vi "VI_read.vi"(8 "error in (no error)":errorcluster, 11 "File bytestream":string) -> (0 "error out":errorcluster, 2 "Resource type":string, 3 "Blocks":T1(c390), 4 "Icon":picture, 5 "Version":T2)   [LabVIEW 2023]
uses:
  <vilib>/Utility/error.llb/Error Cluster From Error Code.vi
  <vilib>/ErrorRing/Error Ring.xnode
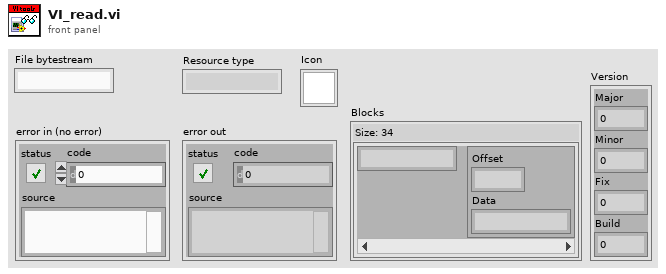
[diagram p1: front panel]
types:
  T1 = map{string, cluster{"Offset":i32, "Data":string}}
  T2 = cluster{"Major":u8, "Minor":u8, "Fix":u8, "Build":u8}
  T3 = cluster{"Int1":u32, "Int2":u32, "Int3":u32, "Offset":u32, "Size":u32}
  T4 = cluster{"RSRC_Identifier":u64, "RSRC_Type":u32, "RSRC_Creator":u32, "Info_Offset":u32, "Info_Size":u32, "Data_Offset":u32, "Data_Size":u32}
  T5 = cluster{"Version":cluster{"Major":u8, "Minor":u8, "Fix":u8, "Build":u8}, "Stage":enum8{"Development", "Alpha", "Beta", "Release"}, "Flags":u16, "VersionString":string, "VersionInfo":string}
  T6 = typedef "imagedata.ctl" = cluster{"image type":i32, "image depth":i32, "image":u8[], "mask":u8[], "colors":u32[], "Rectangle":cluster{"left":i16, "top":i16, "right":i16, "bottom":i16}}
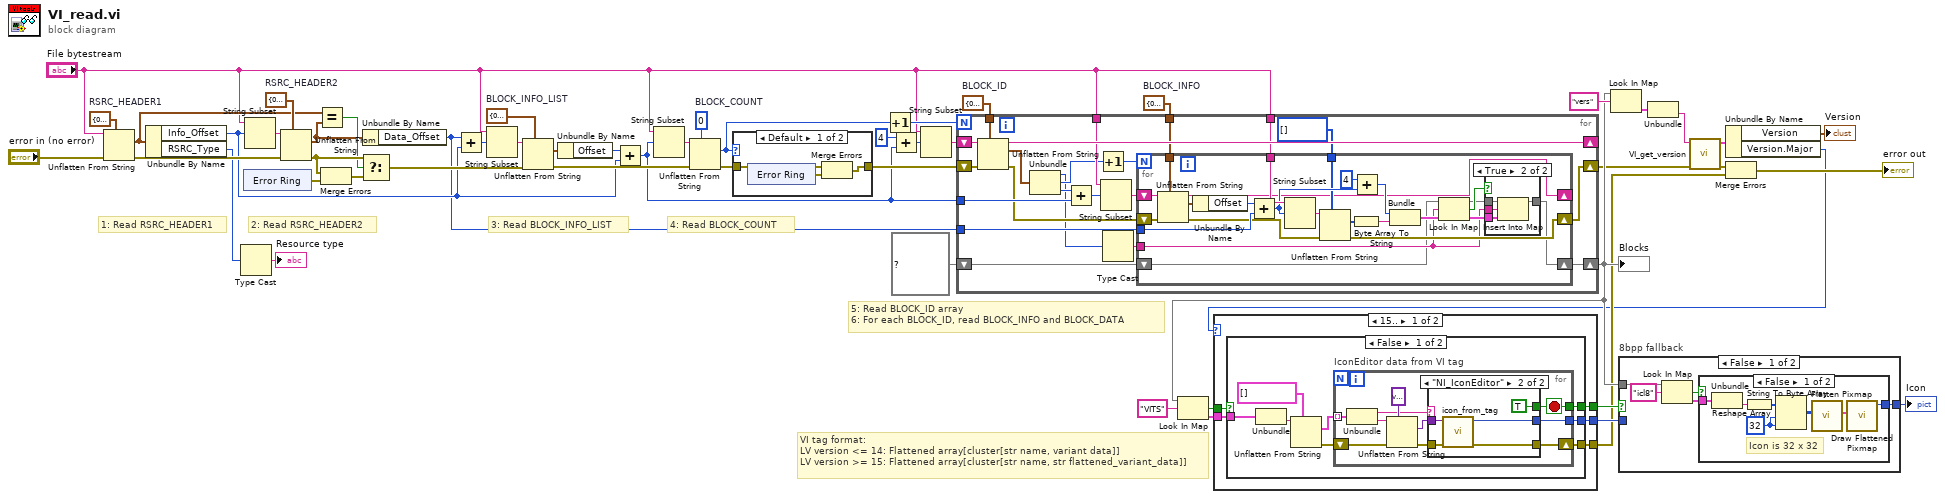
[diagram p0: block diagram]
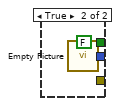
[diagram p3: hidden frame]
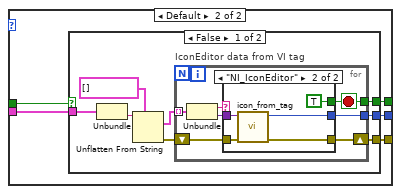
[diagram p4: hidden frame]
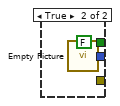
[diagram p6: hidden frame]
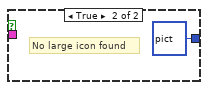
[diagram p7: hidden frame]
diagram:
  w25 = T3 {"Int1"=0, "Int2"=0, "Int3"=0, "Offset"=0, "Size"=0}  # BLOCK_INFO
  w33 = cluster{"Name":u32, "Count":u32, "Offset":u32} {"Name"=0, "Count"=0, "Offset"=0}  # BLOCK_ID
  w37 = 0  # BLOCK_COUNT
  w45 = T3 {"Int1"=0, "Int2"=0, "Int3"=0, "Offset"=0, "Size"=0}  # BLOCK_INFO_LIST
  w47 = T4 {"RSRC_Identifier"=0, "RSRC_Type"=0, "RSRC_Creator"=0, "Info_Offset"=0, "Info_Size"=0, "Data_Offset"=0, "Data_Size"=0}  # RSRC_HEADER2
  w53 = T4 {"RSRC_Identifier"=0, "RSRC_Type"=0, "RSRC_Creator"=0, "Info_Offset"=0, "Info_Size"=0, "Data_Offset"=0, "Data_Size"=0}  # RSRC_HEADER1
  # "VI tag format:\nLV version <= 14: Flattened array[cluster[str name, variant data]]\nLV version >= 15: Flattened array[cluster[str name, str flattened_variant_data]]"
  # "5: Read BLOCK_ID array\n6: For each BLOCK_ID, read BLOCK_INFO and BLOCK_DATA"
  # "4: Read BLOCK_COUNT"
  # "3: Read BLOCK_INFO_LIST"
  # "2: Read RSRC_HEADER2"
  # "1: Read RSRC_HEADER1"
  n1 = Unflatten From String(type=w53, binary string="File bytestream", error in (no error)="error in (no error)") -> (value=w40:T4, error out=w46:errorcluster)  [unwired: 2 in, 1 out]
  n2 = Unbundle By Name(w40) -> ("Info_Offset"=w28:u32, "RSRC_Type"=w20:u32)
  n3 = Type Cast(x=w20) -> (*(type *) &x=→"Resource type":string)  [unwired: 1 in]
  n4 = xnode "Error Ring"() -> ("error out"=w49:errorcluster)
  n5 = String Subset(string="File bytestream", offset (0)=w28) -> (substring=w48:string)  [unwired: 1 in]
  n6 = Unflatten From String(type=w47, binary string=w48, error in (no error)=w46) -> (value=w41:T4, error out=w52:errorcluster)  [unwired: 2 in, 1 out]
  n7 = Equal?(x=w40, y=w41) -> (x = y?=w50:bool)
  n8 = Merge Errors(w52, w49) -> (w51:errorcluster)
  n9 = Select(t=w52, s=w50, f=w51) -> (s? t:f=w42:errorcluster)
  n10 = Unbundle By Name(w41) -> ("Data_Offset"=w24:u32)
  n11 = Add(x=w24, y=w28) -> (x+y=w44:u32)
  n12 = String Subset(string="File bytestream", offset (0)=w44) -> (substring=w43:string)  [unwired: 1 in]
  n13 = Unflatten From String(type=w45, binary string=w43, error in (no error)=w42) -> (value=w35:T3, error out=w34:errorcluster)  [unwired: 2 in, 1 out]
  n14 = Unbundle By Name(w35) -> ("Offset"=w29:u32)
  n15 = Add(x=w29, y=w28) -> (x+y=w22:u32)
  n16 = String Subset(string="File bytestream", offset (0)=w22) -> (substring=w36:string)  [unwired: 1 in]
  n17 = Unflatten From String(type=w37, binary string=w36, error in (no error)=w34) -> (value=w38:i32, error out=w39:errorcluster)  [unwired: 2 in, 1 out]
  n18 = case "Valid Block Count?" shown="Default" w38 {
    tunnel: w39 -> [w55 w61]
    tunnel: [w54 w61] -> w30
    frame Default {
      n19 = xnode "Error Ring"() -> ("error out"=w56:errorcluster)
      n20 = Merge Errors(w55, w56) -> (w54:errorcluster)
    }
    frame 0..1000 {
      # "Valid block count"
    }
  }
  n21 = Increment(x=w38) -> (x+1=w31:i32)
  n22 = Add(x=u32 4 ("value"), y=w22) -> (x+y=w26:u32)
  n23 = String Subset(string="File bytestream", offset (0)=w26) -> (substring=w32:string)  [unwired: 1 in]
  n24 = for {
    N: w31 -> [_]
    shift-right: [w81] -> _
    shift-left: w32 -> [w83]
    tunnel: w33 -> [w82]
    shift-right: [w64] -> w5
    shift-left: w30 -> [w80]
    tunnel: w22 -> [w76]
    tunnel: "File bytestream" -> [w75]
    tunnel: w25 -> [w70]
    tunnel: w24 -> [w69]
    tunnel: "File bytestream" -> [w68]
    shift-right: [w62] -> w6
    shift-left: T1 {} ("map") -> [w63]
    n25 = Unflatten From String(type=w82, binary string=w83, error in (no error)=w80) -> (rest of the binary string=w81:string, value=w74:cluster{"Name":u32, "Count":u32, "Offset":u32}, error out=w71:errorcluster)  [unwired: 2 in]
    n26 = Unbundle(w74) -> ("Name"=w67:u32, "Count"=w73:u32, "Offset"=w72:u32)
    n27 = Add(x=w72, y=w76) -> (x+y=w77:u32)
    n28 = Increment(x=w73) -> (x+1=w79:u32)
    n29 = String Subset(string=w75, offset (0)=w77) -> (substring=w78:string)  [unwired: 1 in]
    n30 = Type Cast(x=w67) -> (*(type *) &x=w66:string)  [unwired: 1 in]
    n31 = for {
      N: w79 -> [_]
      shift-right: [w85] -> _
      shift-left: w78 -> [w106]
      shift-right: [w96] -> w64
      shift-left: w71 -> [w105]
      tunnel: w70 -> [w104]
      tunnel: w69 -> [w103]
      tunnel: w68 -> [w97]
      tunnel: u8[] [] -> [w93]
      tunnel: w66 -> [w87]
      shift-right: [w84] -> w62
      shift-left: w63 -> [w86]
      n32 = Unflatten From String(type=w104, binary string=w106, error in (no error)=w105) -> (rest of the binary string=w85:string, value=w102:T3, error out=w98:errorcluster)  [unwired: 2 in]
      n33 = Unbundle By Name(w102) -> ("Offset"=w101:u32)
      n34 = Add(x=w101, y=w103) -> (x+y=w94:u32)
      n35 = String Subset(string=w97, offset (0)=w94) -> (substring=w100:string)  [unwired: 1 in]
      n36 = Unflatten From String(type=w93, binary string=w100, error in (no error)=w98) -> (value=w99:u8[], error out=w96:errorcluster)  [unwired: 2 in, 1 out]
      n37 = Byte Array To String(unsigned byte array=w99) -> (string=w92:string)
      n38 = Add(x=u32 4 ("value"), y=w94) -> (x+y=w91:u32)
      n39 = Bundle(w91, "string"=w92) -> (w89:cluster{u32, "string":string})  [unwired: 1 in]
      n40 = Look In Map(map=w86, key=w87, default value=w89) -> (key not found?=w90:bool, value=w88:cluster{"Offset":i32, "Data":string})
      n41 = case shown="True" w90 {
        tunnel: w88 -> [_ w111]
        tunnel: w87 -> [_ w110]
        tunnel: w86 -> [w107 w109]
        tunnel: [w107 w108] -> w84
        frame False {
        }
        frame True {
          n42 = Insert Into Map(map in=w109, key=w110, value=w111) -> (map out=w108:T1)  [unwired: 2 out]
        }
      }
    }
  }
  "Blocks" <- w6
  n43 = Look In Map(map=w6, key="VITS") -> (key not found?=w7:bool, value=w11:cluster{"Offset":i32, "Data":string})  [unwired: 1 in]
  n44 = Look In Map(map=w6, key="vers") -> (value=w14:cluster{"Offset":i32, "Data":string})  [unwired: 1 in, 1 out]
  n45 = Unbundle(w14) -> ("Data"=w13:string)  [unwired: 1 out]
  n46 = call "VI_get_version.vi"("error in (no error)"=w5, "vers block"=w13) -> ("error out"=w4:errorcluster, "Version"=w18:T5)  [unwired: 8 in]
  n47 = Unbundle By Name(w18) -> ("Version"=→"Version":T2, "Version.Major"=w1:u8)
  n48 = case shown="15.." w1 {
    tunnel: w11 -> [w116 w147]
    tunnel: [w115 w146] -> w9
    tunnel: [w114 w145] -> w8
    tunnel: w7 -> [w113 w144]
    tunnel: [w112 w143] -> w3
    frame 15.. {
      n49 = case shown="False" w113 {
        tunnel: w116 -> [w124 _]
        tunnel: [w119 FALSE] -> w115
        tunnel: [w118 w142] -> w114
        tunnel: [w117 _] -> w112
        frame False {
          n50 = Unbundle(w124) -> ("Data"=w120:string)  [unwired: 1 out]
          n51 = Unflatten From String(type=cluster{"Tag":string, "Data":string}[] [] ("Tags"), binary string=w120) -> (value=w121:cluster{"Tag":string, "Data":string}[], error out=w123:errorcluster)  [unwired: 3 in, 1 out]
          n52 = for "IconEditor data from VI tag" {
            tunnel: w121 -> [w132] mode=indexing
            shift-right: [w127] -> w117
            shift-left: w123 -> [w134]
            tunnel: [w126] -> w119
            tunnel: [w125] -> w118
            stop <- w126 stop-if-true
            n53 = Unbundle(w132) -> ("Tag"=w129:string, "Data"=w131:string)
            n54 = Unflatten From String(type=variant, binary string=w131, error in (no error)=w134) -> (value=w130:variant, error out=w128:errorcluster)  [unwired: 2 in, 1 out]
            n55 = case shown="\"NI_IconEditor\"" w129 {
              tunnel: w130 -> [_ w139]
              tunnel: [_ w138] -> w125
              tunnel: [_ TRUE] -> w126
              tunnel: w128 -> [w135 w137]
              tunnel: [w135 w136] -> w127
              frame "False", Default {
              }
              frame "NI_IconEditor" {
                n56 = call "icon_from_tag.vi"("error in (no error)"=w137, "Tag in"=w139) -> ("error out"=w136:errorcluster, "Icon"=w138:picture)  [unwired: 8 in]
              }
            }
          }
        }
        frame True {
          n57 = call "Empty Picture"() -> ("empty picture"=w142:picture)
        }
      }
    }
    frame Default {
      n58 = case shown="False" w144 {
        tunnel: w147 -> [w155 _]
        tunnel: [w151 FALSE] -> w146
        tunnel: [w150 w170] -> w145
        tunnel: [w149 _] -> w143
        frame False {
          n59 = Unbundle(w155) -> ("Data"=w152:string)  [unwired: 1 out]
          n60 = Unflatten From String(type=cluster{"Tag":string, "Data":variant}[] [] ("Tags"), binary string=w152) -> (value=w153:cluster{"Tag":string, "Data":variant}[], error out=w154:errorcluster)  [unwired: 3 in, 1 out]
          n61 = for "IconEditor data from VI tag" {
            tunnel: w153 -> [w162] mode=indexing
            shift-right: [w160] -> w149
            shift-left: w154 -> [w156]
            tunnel: [w159] -> w151
            tunnel: [w158] -> w150
            stop <- w159 stop-if-true
            n62 = Unbundle(w162) -> ("Tag"=w161:string, "Data"=w157:variant)
            n63 = case shown="\"NI_IconEditor\"" w161 {
              tunnel: w157 -> [_ w167]
              tunnel: [_ w166] -> w158
              tunnel: [_ TRUE] -> w159
              tunnel: w156 -> [w163 w165]
              tunnel: [w163 w164] -> w160
              frame "False", Default {
              }
              frame "NI_IconEditor" {
                n64 = call "icon_from_tag.vi"("error in (no error)"=w165, "Tag in"=w167) -> ("error out"=w164:errorcluster, "Icon"=w166:picture)  [unwired: 8 in]
              }
            }
          }
        }
        frame True {
          n65 = call "Empty Picture"() -> ("empty picture"=w170:picture)
        }
      }
    }
  }
  n66 = case "8bpp fallback" shown="False" w9 {
    tunnel: w8 -> [_ w184]
    tunnel: [w175 w184] -> w12
    tunnel: w6 -> [w173 _]
    frame False {
      n67 = Look In Map(map=w173, key="icl8") -> (key not found?=w172:bool, value=w174:cluster{"Offset":i32, "Data":string})  [unwired: 1 in]
      n68 = case shown="False" w172 {
        tunnel: [w178 picture bytes[3102] ("no icon")] -> w175
        tunnel: w174 -> [w177 _]
        frame False {
          w179 = 32 ("dimension size")
          # "Icon is 32 x 32"
          n69 = Unbundle(w177) -> ("Data"=w176:string)  [unwired: 1 out]
          n70 = String To Byte Array(string=w176) -> (unsigned byte array=w181:u8[])
          n71 = Reshape Array(w181, w179, w179) -> (w180:u8[][])
          n72 = call <vilib>:"Flatten Pixmap.vi"("8-bit pixmap"=w180) -> ("image data"=w182:T6)  [unwired: 5 in, 5 out]
          n73 = call <vilib>:"Draw Flattened Pixmap.vi"("image data"=w182) -> ("new picture"=w178:picture)  [unwired: 1 in, 7 out]
        }
        frame True {
          # "No large icon found"
        }
      }
    }
    frame True {
    }
  }
  "Icon" <- w12
  n74 = Merge Errors(w4, w3) -> (→"error out":errorcluster)
